vi "Is output settled.vi"(8 "error in (no error)":errorcluster, 11 "Source in":refnum<class "Source.lvclass">) -> (0 "error out":errorcluster, 2 "Is settled?":bool, 3 "Source out":refnum<class "Source.lvclass">)   [LabVIEW 2015, in "Source.lvclass"]
uses:
  Source.lvclass
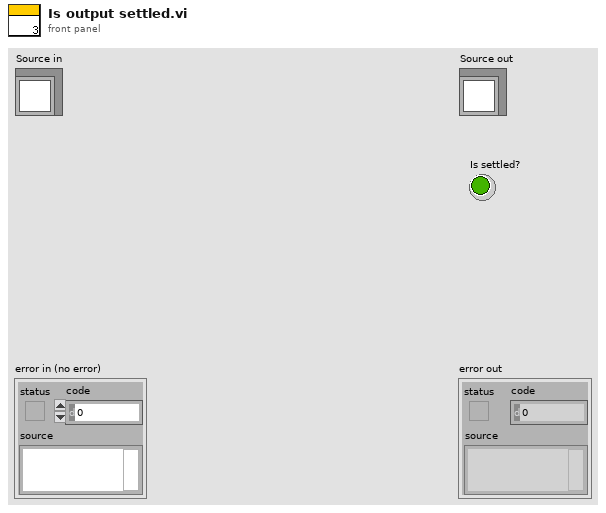
[diagram p1: front panel]
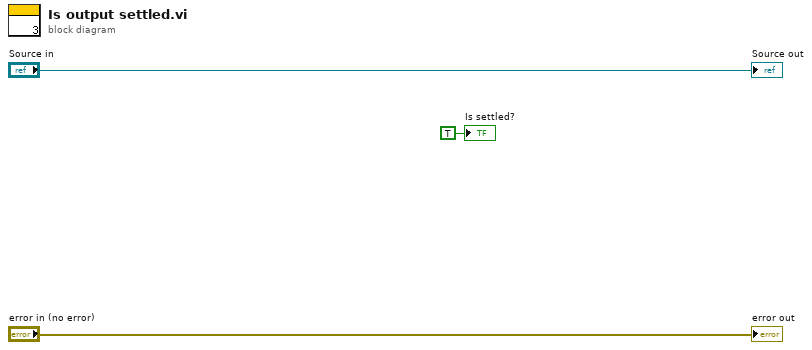
[diagram p0: block diagram]
diagram:
  "error out" <- "error in (no error)"
  "Source out" <- "Source in"
  "Is settled?" <- TRUE ("Is settled?")
